vi "Configure Sequence Condition.vi"(6 "Reset Condition (No Reset)":string(combo)="NONE,NONE,NONE", 8 "error in (no error)":errorcluster {"code" format="%.0x"}, 9 "Trigger Condition (Pattern2 Entered)":string(combo)="PATT2,ENT,NONE", 10 "Find Condition (Pattern1 Entered)":string(combo)="PATT1,ENT,NONE", 11 "VISA Resource Name":refnum<visa-resource-name>) -> (0 "error out":errorcluster {"code" format="%.0x"}, 3 "VISA Resource Name Out":refnum<visa-resource-name>)   [LabVIEW 2011, in "Agilent 546XX Series.lvlib"]
doc: "This VI configures the find stage, trigger on stage, and reset on stage conditions.\n\nNote: This VI affects instrument behavior only if the trigger type is set to Sequence. Call the ag546xx Configure Trigger and ag546xx Configure Trigger Coupling VIs to set the trigger type and trigger coupling before calling this VI."
uses:
  Agilent 546XX Series.lvlib
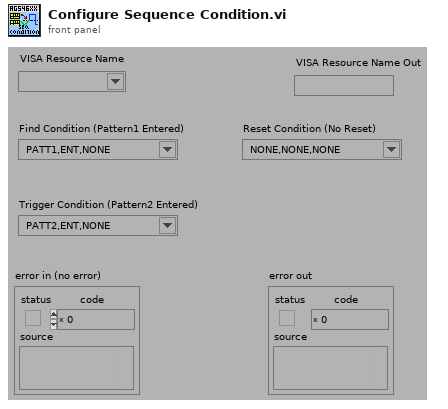
[diagram p1: front panel]
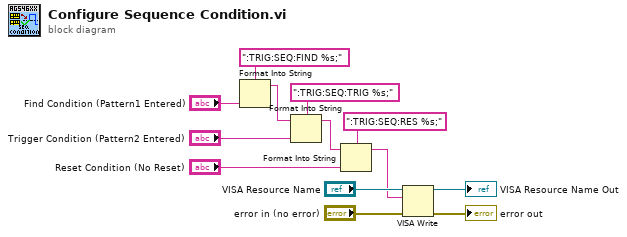
[diagram p0: block diagram]
diagram:
  n1 = Format Into String(format string=":TRIG:SEQ:FIND %s;", "Find Condition (Pattern1 Entered)") -> (resulting string=w7:string)  [unwired: 2 in, 1 out]
  n2 = Format Into String(format string=":TRIG:SEQ:TRIG %s;", initial string=w7, "Trigger Condition (Pattern2 Entered)") -> (resulting string=w3:string)  [unwired: 1 in, 1 out]
  n3 = Format Into String(format string=":TRIG:SEQ:RES %s;", initial string=w3, "Reset Condition (No Reset)") -> (resulting string=w1:string)  [unwired: 1 in, 1 out]
  n4 = VISA Write(VISA resource name="VISA Resource Name", write buffer=w1, error in (no error)="error in (no error)") -> (VISA resource name out=→"VISA Resource Name Out":refnum<visa-resource-name>, error out=→"error out":errorcluster)  [unwired: 1 out]
